vi "Assignment_01_OPT.vi"() -> ()   [LabVIEW 2023]
panel:
  in  "Stop":bool
  out "B":i32
  out "A":i32
  in  "Tab Control":enum32{"Page 1", "Page 2", "Page 3", "Page 4"}(tab)
  in  "N1":i32
  in  "N2":i32
  in  "N3":i32=4
  in  "N4":i32=2
  in  "N5":i32
  in  "N6":i32
  in  "N7":i32
  in  "N8":i32
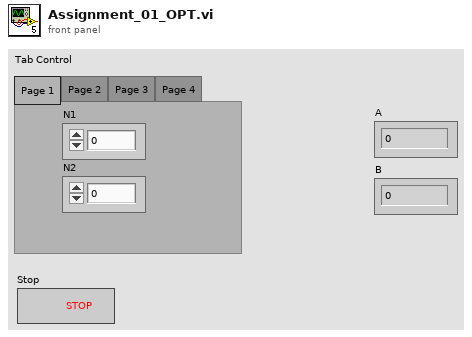
[diagram p1: front panel]
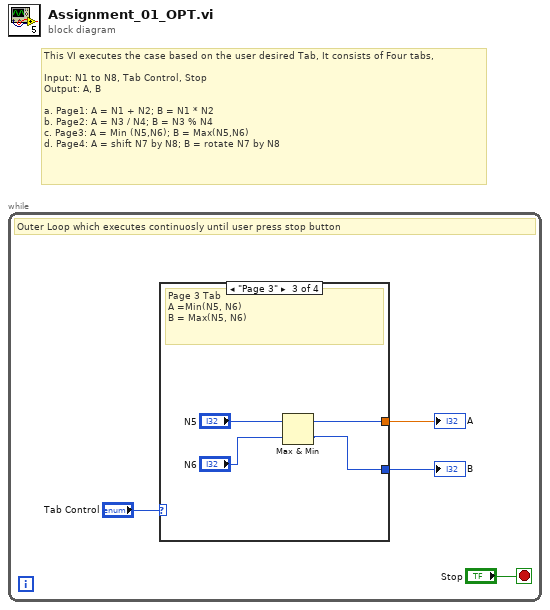
[diagram p0: block diagram]
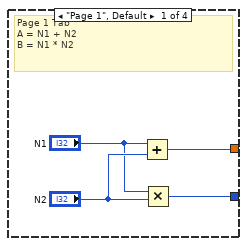
[diagram p2: hidden frame]
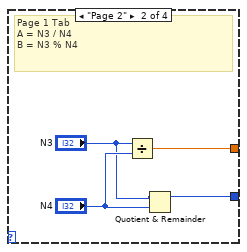
[diagram p3: hidden frame]
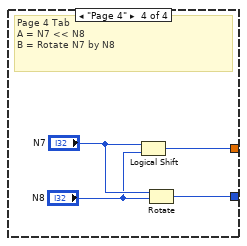
[diagram p4: hidden frame]
diagram:
  # "This VI executes the case based on the user desired Tab, It consists of Four tabs,\n\nInput: N1 to N8, Tab Control, Stop\nOutput: A, B\n\na. Page1: A = N1 + N2; B = N1 * N2\nb. Page2: A = N3 / N4; B = N3 % N4 \nc. Page3: A = Min (N5,N6); B = Max(N5,N6)\nd. Page4: A = shift N7 by N8; B = rotate N7 by N8"
  n1 = while {
    stop <- "Stop" stop-if-true
    # "Outer Loop which executes continuosly until user press stop button"
    n2 = case shown="\"Page 3\"" "Tab Control" {
      tunnel: [w8 w12 w16 w17] -> w3
      tunnel: [w5 w9 w15 w20] -> w2
      frame "Page 1", Default {
        # "Page 1 Tab\nA = N1 + N2\nB = N1 * N2"
        n3 = Add(x="N1", y="N2") -> (x+y=w8:i32)
        n4 = Multiply(x="N1", y="N2") -> (x*y=w5:i32)
      }
      frame "Page 2" {
        # "Page 1 Tab\nA = N3 / N4\nB = N3 % N4"
        n5 = Divide(x="N3", y="N4") -> (x/y=w12:dbl)
        n6 = Quotient & Remainder(x="N3", y="N4") -> (x-y*floor(x/y)=w9:i32)  [unwired: 1 out]
      }
      frame "Page 3" {
        # "Page 3 Tab\nA =Min(N5, N6)\nB = Max(N5, N6)"
        n7 = Max & Min(x="N5", y="N6") -> (max(x,y)=w16:i32, min(x,y)=w15:i32)
      }
      frame "Page 4" {
        # "Page 4 Tab\nA = N7 << N8\nB = Rotate N7 by N8"
        n8 = Logical Shift(y="N7", x="N8") -> (x << y=w17:i32)
        n9 = Rotate(1:"N8", 2:"N7") -> (0:w20:i32)
      }
    }
    "A" <- w3
    "B" <- w2
  }
